vi "X.vi"(11 "DataIn":T4) -> (3 "DataOut":T1)   [LabVIEW 2017]
doc: "SubVI criada para mostrar popup para o usuário indicando que o player X foi o vencedor."
uses:
  controls/DataIn.ctl
  controls/Tabuleiro.ctl
  controls/GameOption.ctl
  controls/DataOut.ctl
panel:
  in  "ok":bool
  # "X é o vencedor!"
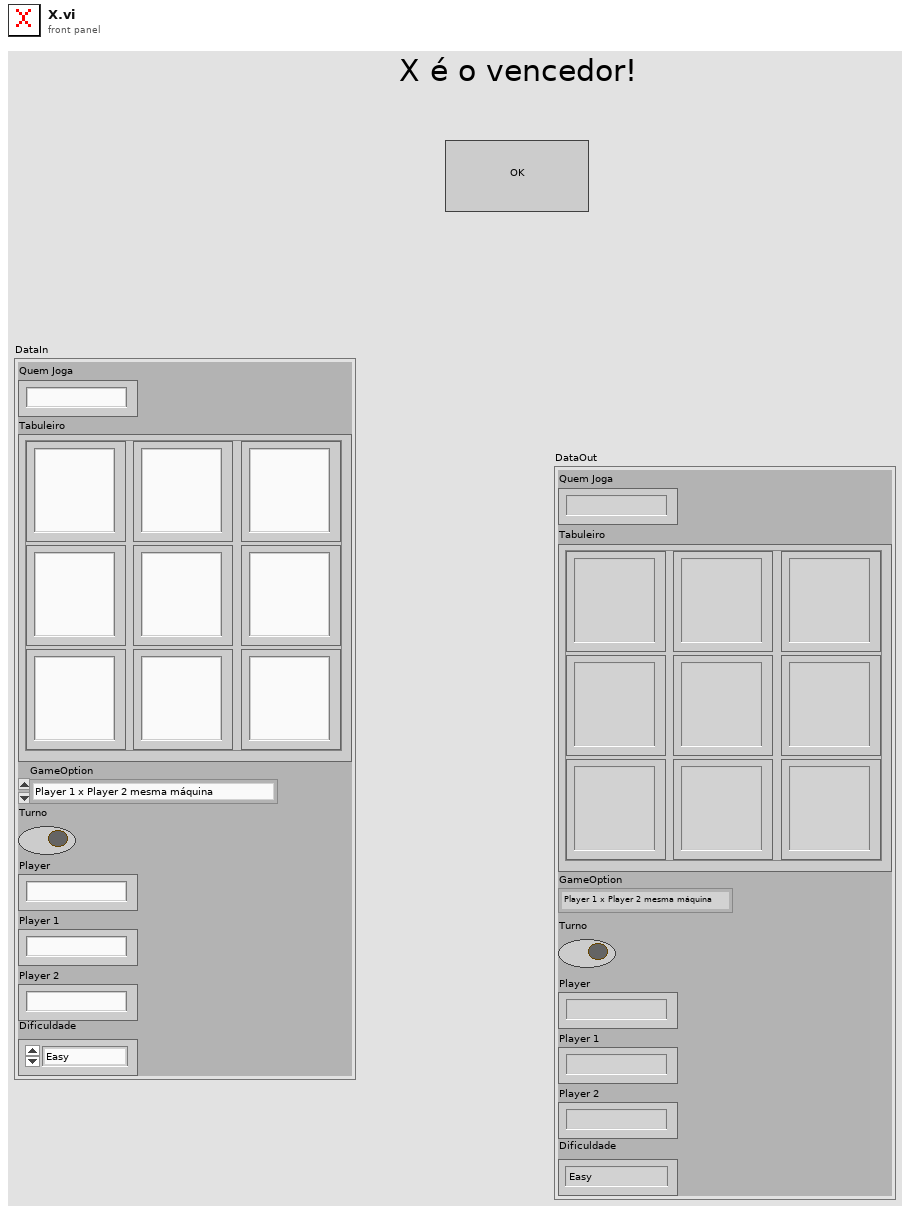
[diagram p1: front panel]
types:
  T1 = typedef "DataOut.ctl" = cluster{"Quem Joga":string, "Tabuleiro":T2, "GameOption":T3, "Turno":bool, "Player":string, "Player 1":string, "Player 2":string, "Dificuldade":enum16{"Easy", "Medium", "Hard"}}
  T2 = typedef "Tabuleiro.ctl" = cluster{"(0,0)":string, "(1,0)":string, "(0,1)":string, "(1,1)":string, "(2,0)":string, "(1,2)":string, "(2,2)":string, "(0,2)":string, "(2,1) ":string}
  T3 = typedef "GameOption.ctl" = enum16{"Player 1 x Player 2 mesma máquina", "Player 1 x Player 2 pela rede", "Player 1 x Computador", "Wait for Event", "Initialize"}
  T4 = typedef "DataIn.ctl" = cluster{"Quem Joga":string, "Tabuleiro":T2, "GameOption":T3, "Turno":bool, "Player":string, "Player 1":string, "Player 2":string, "Dificuldade":enum16{"Easy", "Medium", "Hard"}}
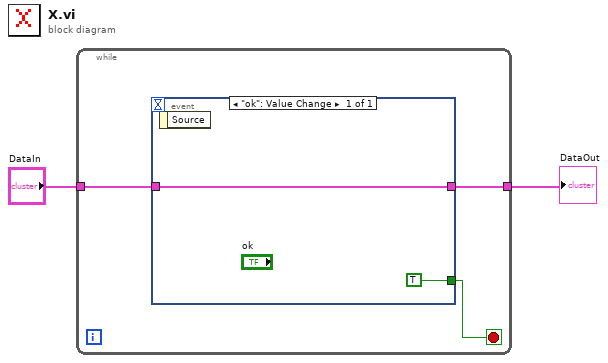
[diagram p0: block diagram]
diagram:
  n1 = while {
    tunnel: "DataIn" -> [w4]
    tunnel: [w5] -> w1
    stop <- w3 stop-if-true
    n2 = event shown="[0] \"ok\": Value Change" {
      selector: _ -> [_]
      dyn-events: _ -> [_]
      timeout: _ -> [_]
      tunnel: [w7] -> w5
      tunnel: w4 -> [w7]
      tunnel: [TRUE] -> w3
      event "ok": Value Change {
        n3 = event-data() -> ()  [unwired: 1 in, 1 out]
      }
    }
  }
  "DataOut" <- w1
